vi "Check for missing VIs on LV project.vi"(8 "error in (no error)":errorcluster) -> (0 "error out":errorcluster, 3 "Pass":bool)   [LabVIEW 2021]
panel:
  out "Array":path[](array[path])
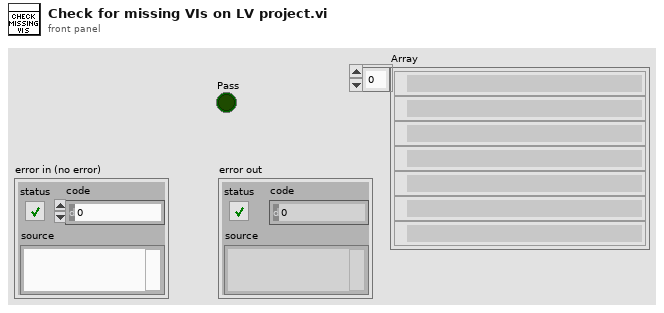
[diagram p1: front panel]
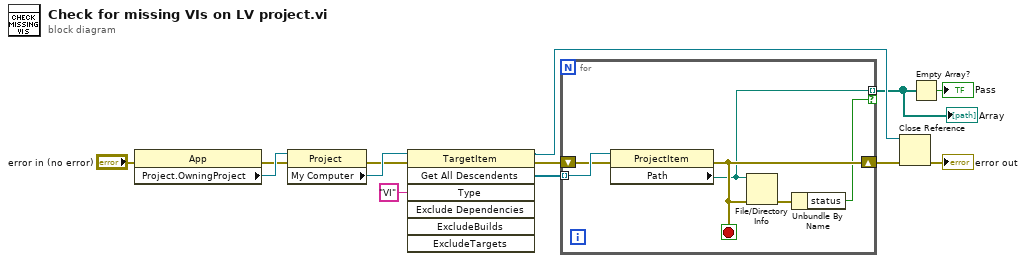
[diagram p0: block diagram]
diagram:
  n1 = property class="App"(error in="error in (no error)") -> (error out=w8:errorcluster, "Project.OwningProject"=w13:refnum<vi>)  [unwired: 1 in, 1 out]
  n2 = property class="Project"(reference=w13, error in=w8) -> (error out=w9:errorcluster, "My Computer"=w12:refnum<vi>)  [unwired: 1 out]
  n3 = invoke class="TargetItem" method="Get All Descendents"(reference=w12, error in=w9, "Type"="VI") -> (reference out=w5:refnum<vi>, error out=w7:errorcluster, "All Descendents"=w10:refnum<vi>[])  [unwired: 4 in, 4 out]
  n4 = for {
    tunnel: w10 -> [w19] mode=indexing
    shift-right: [w16] -> w6
    shift-left: w7 -> [w18]
    tunnel: [w15] -> w2 mode=indexing if=w14
    stop <- w16 stop-if-true
    n5 = property class="ProjectItem"(reference=w19, error in=w18) -> (error out=w16:errorcluster, "Path"=w15:path)  [unwired: 1 out]
    n6 = File/Directory Info(path=w15, error in=w16) -> (error out=w17:errorcluster)  [unwired: 6 out]
    n7 = Unbundle By Name(w17) -> ("status"=w14:bool)
  }
  "Array" <- w2
  n8 = Close Reference(reference=w5, error in (no error)=w6) -> (error out=→"error out":errorcluster)
  n9 = Empty Array?(array=w2) -> (empty?=→"Pass":bool)
